vi "Particle Filter_calib.vi"(6 "Range":cluster{"Lower value":sgl, "Upper value":sgl}={"Lower value"=40.0, "Upper value"=255.0}, 8 "error in":errorcluster, 11 "Source Image":T1(plugin-control) caption="Original Image") -> (0 "error out":errorcluster, 2 "Location in Pixels":T2(array[cluster]), 3 "Ref Image (8 bit)":T1)   [LabVIEW 2020]
doc: "This example performs a series of grayscale filtering, threshold, binary morphology, and particle analysis operations to measure the areas of all the large circular particles of the image."
uses:
  <vilib>/vision/Image Controls.llb/IMAQ Image.ctl
  <vilib>/vision/NI_Vision_Development_Module.lvlib
panel:
  in  "Source Image 2":T1(plugin-control) caption="Original Image"
  in  "Tab Control":T3(tab)
  out "Threshold":T1(plugin-control) caption="Threshold Image"
  out "Fill Hole and Reject Border":T1(plugin-control) caption="Reject Border and Fill Holes"
  out "Filter and Overlay Area":T1(plugin-control) caption="Filter Out Non Circles and Overlay Particle Area"
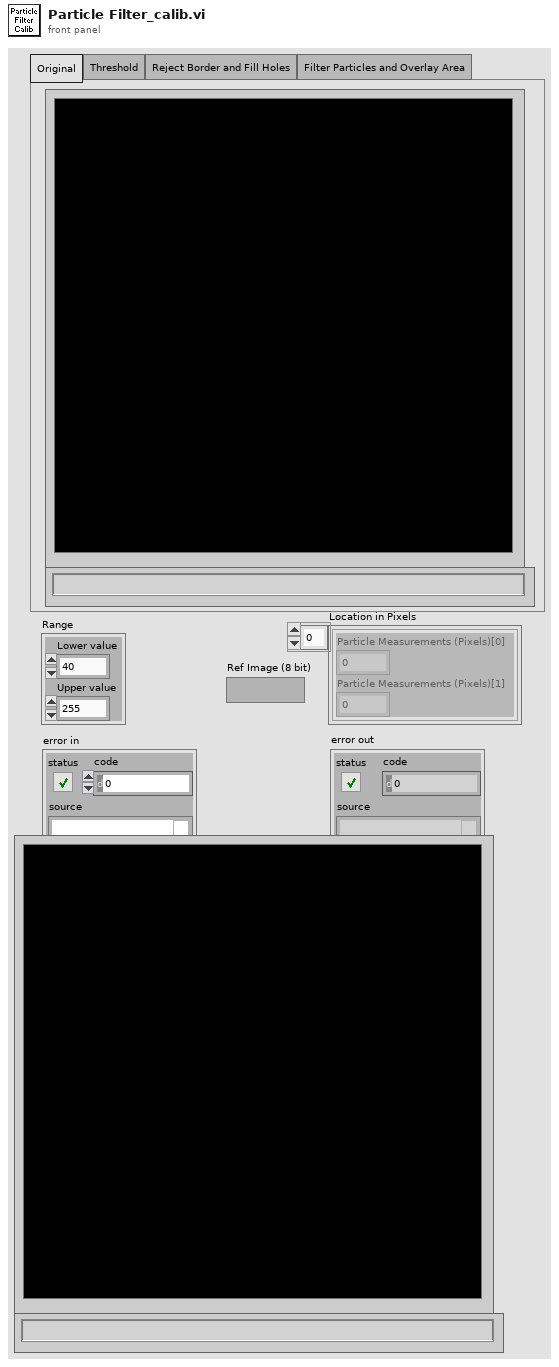
[diagram p1: front panel]
types:
  T1 = typedef "IMAQ Image.ctl" = refnum<image>
  T2 = cluster{"Particle Measurements (Pixels)[0]":dbl, "Particle Measurements (Pixels)[1]":dbl}[]
  T3 = enum32{"Original", "Threshold", "Reject Border and Fill Holes", "Filter Particles and Overlay Area"}
  T4 = typedef "Image Type" = u32
  T5 = typedef "Particle Parameters" = i32
  T6 = cluster{"Measurement Parameter":T5, "Range Lower Value":dbl, "Range Upper Value":dbl, "Range":bool, "Measurement Type":bool}[]
  T7 = cluster{"Desired Font (Application)":enum16{"User-specified Font", "Application Font", "System Font", "Dialog Font"}, "[User-specified Font]":cluster{"Font Name":string, "Size":i16, "Strikeout?":bool, "Italic?":bool, "Underline?":bool, "Outline?":bool, "Shadow?":bool, "Bold?":bool, "Rotation Angle":dbl}, "Horizontal Alignment":i16, "Vertical Alignment":i16}
  T8 = cluster{"Particle Measurements (Pixels)[0]":dbl, "Particle Measurements (Pixels)[1]":dbl, "Particle Measurements (Pixels)[2]":dbl}
  T9 = cluster{"Particle Measurements (Pixels)[0]":dbl, "Particle Measurements (Pixels)[1]":dbl}
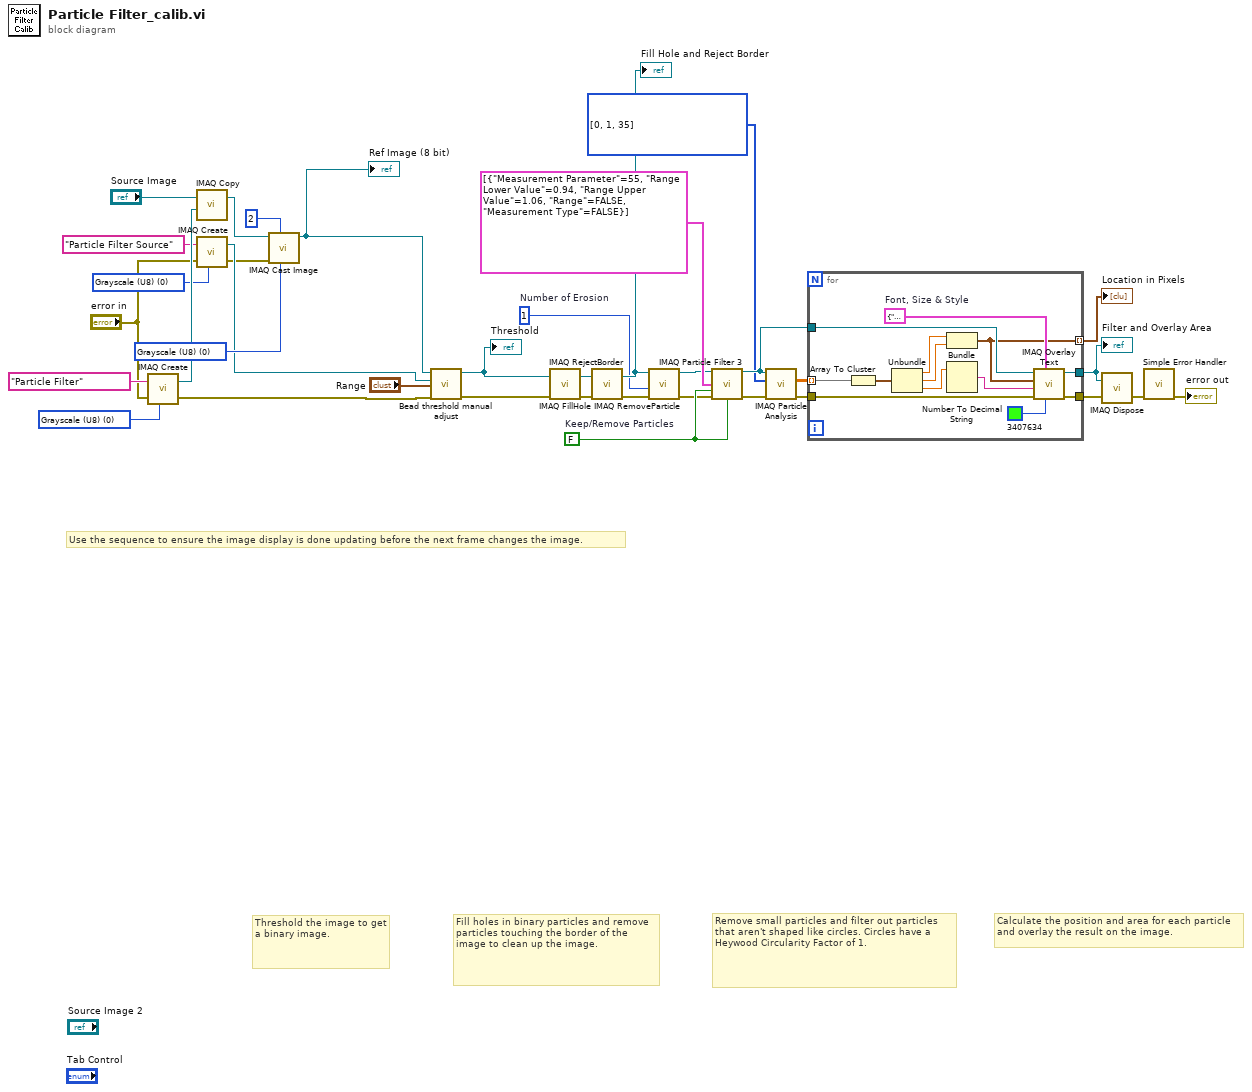
[diagram p0: block diagram]
diagram:
  w5 = T4 0 items=["Grayscale (U8)", "Grayscale (I16)", "Grayscale (SGL)", "Complex (CSG)", "RGB (U32)", "HSL (U32)", "RGB (U64)", "Grayscale (U16)"] ("Image Type")
  w12 = T4 0 items=["Grayscale (U8)", "Grayscale (I16)", "Grayscale (SGL)", "Complex (CSG)", "RGB (U32)", "HSL (U32)", "RGB (U64)", "Grayscale (U16)"] ("Image Type")
  w13 = T4 0 items=["Grayscale (U8)", "Grayscale (I16)", "Grayscale (SGL)", "Complex (CSG)", "RGB (U32)", "HSL (U32)", "RGB (U64)", "Grayscale (U16)"] ("Image Type")
  w17 = 1  # Number of Erosion
  w19 = FALSE  # Keep/Remove Particles
  w20 = T5[] [0, 1, 35] items=["Center of Mass X", "Center of Mass Y", "First Pixel X", "First Pixel Y", "Bounding Rect Left", "Bounding Rect Top", "Bounding Rect Right", "Bounding Rect Bottom", "Max Feret Diameter Start X", "Max Feret Diameter Start Y", "Max Feret Diameter End X", "Max Feret Diameter End Y", "Max Horiz. Segment Length Left", "Max Horiz. Segment Length Right", "Max Horiz. Segment Length Row", "-", "Bounding Rect Width", "Bounding Rect Height", "Bounding Rect Diagonal", "Perimeter", "Convex Hull Perimeter", "Holes' Perimeter", "Max Feret Diameter", "Equivalent Ellipse Major Axis", "Equivalent Ellipse Minor Axis", "Equivalent Ellipse Minor Axis (Feret)", "Equivalent Rect Long Side", "Equivalent Rect Short Side", "Equivalent Rect Diagonal", "Equivalent Rect Short Side (Feret)", "Average Horiz. Segment Length", "Average Vert. Segment Length", "Hydraulic Radius", "Waddel Disk Diameter", "-", "Area", "Holes' Area", "Particle & Holes' Area", "Convex Hull Area", "Image Area", "-", "Number of Holes", "Number of Horiz. Segments", "Number of Vert. Segments", "-", "Orientation", "Max Feret Diameter Orientation", "-", "% Area/Image Area", "% Area/(Particle & Holes' Area)", "Ratio of Equivalent Ellipse Axes", "Ratio of Equivalent Rect Sides", "-", "Elongation Factor", "Compactness Factor", "Heywood Circularity Factor", "Type Factor", "-", "Sum X", "Sum Y", "Sum XX", "Sum XY", "Sum YY", "Sum XXX", "Sum XXY", "Sum XYY", "Sum YYY", "-", "Moment of Inertia XX", "Moment of Inertia XY", "Moment of Inertia YY", "Moment of Inertia XXX", "Moment of Inertia XXY", "Moment of Inertia XYY", "Moment of Inertia YYY", "Norm. Moment of Inertia XX", "Norm. Moment of Inertia XY", "Norm. Moment of Inertia YY", "Norm. Moment of Inertia XXX", "Norm. Moment of Inertia XXY", "Norm. Moment of Inertia XYY", "Norm. Moment of Inertia YYY", "Hu Moment 1", "Hu Moment 2", "Hu Moment 3", "Hu Moment 4", "Hu Moment 5", "Hu Moment 6", "Hu Moment 7"] ("Pixel Measurements")
  # "Calculate the position and area for each particle and overlay the result on the image."
  # "Remove small particles and filter out particles that aren't shaped like circles. Circles have a Heywood Circularity Factor of 1."
  # "Fill holes in binary particles and remove particles touching the border of the image to clean up the image."
  # "Threshold the image to get a binary image."
  # "Use the sequence to ensure the image display is done updating before the next frame changes the image."
  n1 = call "IMAQ Create"("Image Name"="Particle Filter", "Image Type"=w12, "error in (no error)"="error in") -> ("New Image"=w8:T1, "error out"=w11:errorcluster)  [unwired: 2 in]
  n2 = call "IMAQ Copy"("Image Dst"=w8, "Image Src"="Source Image") -> ("Image Dst Out"=w7:T1)  [unwired: 4 in, 1 out]
  n3 = call "IMAQ Create"("Image Name"="Particle Filter Source", "Image Type"=w5, "error in (no error)"="error in") -> ("New Image"=w3:T1, "error out"=w1:errorcluster)  [unwired: 2 in]
  n4 = call "IMAQ Cast Image"("Image Type"=w13, "# Shifts"=2, "error in (no error)"=w1, "Image Src"=w7) -> ("Image Dst Out"=w10:T1)  [unwired: 6 in, 1 out]
  "Ref Image (8 bit)" <- w10
  n5 = call "Bead threshold manual adjust.vi"("error in (no error)"=w11, "Range"="Range", "Particle Filter Image"=w3, "Image Source"=w10) -> ("error out"=w31:errorcluster, "Refnum out"=w32:T1)  [unwired: 6 in]
  "Threshold" <- w32
  n6 = call "IMAQ FillHole"("error in (no error)"=w31, "Image Src"=w32) -> ("error out"=w25:errorcluster, "Image Dst Out"=w26:T1)  [unwired: 4 in]
  n7 = call "IMAQ RejectBorder"("error in (no error)"=w25, "Image Src"=w26) -> ("error out"=w30:errorcluster, "Image Dst Out"=w29:T1)  [unwired: 4 in]
  "Fill Hole and Reject Border" <- w29
  n8 = call "IMAQ RemoveParticle"("error in (no error)"=w30, "Number of Erosion"=w17, "Image Src"=w29) -> ("error out"=w15:errorcluster, "Image Dst Out"=w16:T1)  [unwired: 7 in]
  n9 = call "IMAQ Particle Filter 3"("Image Src"=w16, "Selection Values"=T6 [{"Measurement Parameter"=55, "Range Lower Value"=0.94, "Range Upper Value"=1.06, "Range"=FALSE, "Measurement Type"=FALSE}], "Keep/Remove Particles (F)"=w19, "error in (no error)"=w15, "Fill Holes? (F)"=w19) -> ("Image Dst Out"=w23:T1, "error out"=w24:errorcluster)  [unwired: 8 in, 1 out]
  n10 = call "IMAQ Particle Analysis"("error in (no error)"=w24, "Pixel Measurements"=w20, "Image"=w23) -> ("error out"=w21:errorcluster, "Particle Measurements (Pixels)"=w22:dbl[][])  [unwired: 3 in, 4 out]
  n11 = for {
    tunnel: w21 -> [w49]
    tunnel: [w48] -> w28
    tunnel: [w47] -> w27
    tunnel: w23 -> [w44]
    tunnel: w22 -> [w39] mode=indexing
    tunnel: [w37] -> w33 mode=indexing
    w38 = T7 {"Desired Font (Application)"=enum."Application Font", "[User-specified Font]"={"Font Name"="", "Size"=12, "Strikeout?"=FALSE, "Italic?"=FALSE, "Underline?"=FALSE, "Outline?"=FALSE, "Shadow?"=FALSE, "Bold?"=FALSE, "Rotation Angle"=0.0}, "Horizontal Alignment"=0, "Vertical Alignment"=0}  # Font, Size & Style
    n12 = Array To Cluster(array=w39) -> (cluster=w43:T8)
    n13 = Unbundle(w43) -> ("Particle Measurements (Pixels)[0]"=w42:dbl, "Particle Measurements (Pixels)[1]"=w41:dbl, "Particle Measurements (Pixels)[2]"=w40:dbl)
    n14 = Bundle("Particle Measurements (Pixels)[0]"=w42, "Particle Measurements (Pixels)[1]"=w41) -> (w37:T9)  [unwired: 1 in]
    n15 = Number To Decimal String(number=w40) -> (decimal integer string=w46:string)  [unwired: 1 in]
    n16 = call "IMAQ Overlay Text"("Text Color (black)"=u32 3407634, "Font, Size & Style"=w38, "error in (no error)"=w49, "String"=w46, "Origin"=w37, "Image"=w44) -> ("error out"=w48:errorcluster, "Image Out"=w47:T1)  [unwired: 4 in]
  }
  "Location in Pixels" <- w33
  "Filter and Overlay Area" <- w27
  n17 = call "IMAQ Dispose"("Image"=w27, "error in (no error)"=w28) -> ("error out"=w14:errorcluster)  [unwired: 4 in]
  n18 = call <vilib>:"Simple Error Handler.vi"("error in (no error)"=w14) -> ("error out"=→"error out":errorcluster)  [unwired: 4 in, 4 out]
